vi "Get Service.vi"(8 "error in (no error)":errorcluster, 10 "Class Name":string, 11 "Server in":refnum<class "Server.lvclass">) -> (0 "error out":errorcluster, 2 "Service.lvclass":refnum<class "Service.lvclass">, 3 "Server out":refnum<class "Server.lvclass">)   [LabVIEW 2024, in "Ramses Framework.lvlib" / "Server.lvclass"]
uses:
  Server.lvclass
  Service/Service.lvclass
  Server.lvclass/Server.ctl
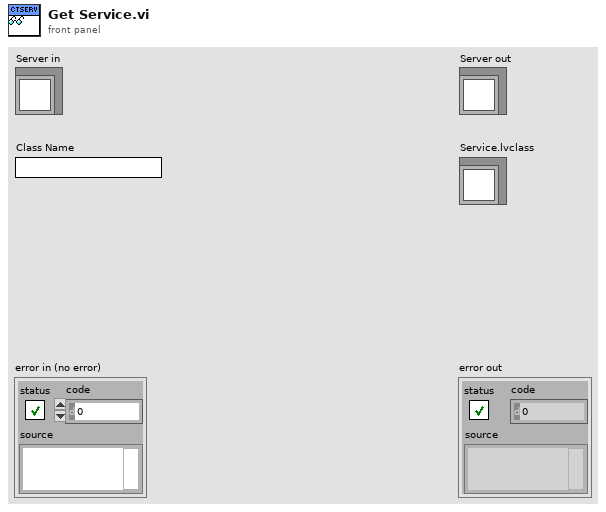
[diagram p1: front panel]
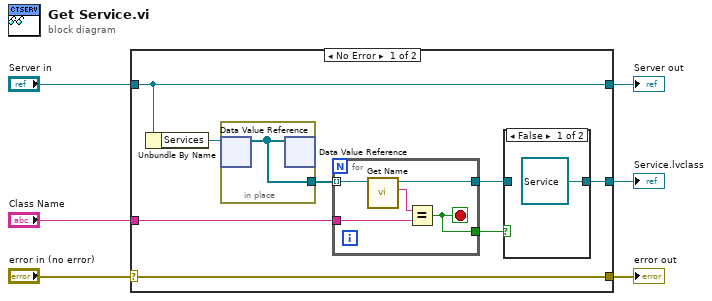
[diagram p0: block diagram]
diagram:
  n1 = case shown="No Error" "error in (no error)" {
    selector: "error in (no error)" -> [w14 w23]
    tunnel: [w14 w23] -> w5
    tunnel: [w13 w24] -> w3
    tunnel: "Server in" -> [w13 w24]
    tunnel: [w10 _] -> w2
    tunnel: "Class Name" -> [w12 _]
    frame No Error {
      n2 = Unbundle By Name(w13) -> ("Services"=w8:refnum<data-value>)
      n3 = in-place {
        in-place-border: [w15] -> w7
        n4 = in-place-dvr #1(w8) -> (w15:refnum<class "Service.lvclass">[])  [unwired: 1 out]
        n5 = in-place-dvr #1(w15) -> ()  [unwired: 2 out]
      }
      n6 = for {
        tunnel: w7 -> [w22] mode=indexing
        tunnel: w12 -> [w20]
        tunnel: [w19] -> w9
        tunnel: [w18] -> w11
        stop <- w18 stop-if-true
        n7 = call "Get Name.vi"("Service in"=w22) -> ("Name"=w21:string, "Service out"=w19:refnum<class "Service.lvclass">)  [unwired: 8 in, 1 out]
        n8 = Equal?(x=w21, y=w20) -> (x = y?=w18:bool)
      }
      n9 = case shown="False" w11 {
        tunnel: [refnum<class "Service.lvclass"> refnum ("Service out") w17] -> w10
        tunnel: w9 -> [_ w17]
        frame False {
        }
        frame True {
        }
      }
    }
    frame Error {
    }
  }
  "error out" <- w5
  "Server out" <- w3
  "Service.lvclass" <- w2
